vi "CheckTracepoint.vi"(8 "error in (no error)":errorcluster, 11 "tracepoint":string) -> (0 "error out":errorcluster, 1 "found":bool, 2 "enabled":bool)   [LabVIEW 2017, in "TraceLogger.lvlib"]
uses:
  <vilib>/addons/TraceLogger/TraceLogger.lvlib
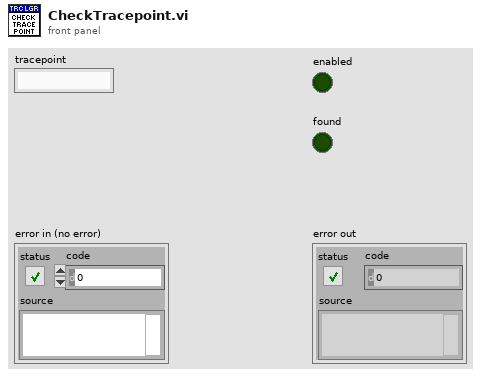
[diagram p1: front panel]
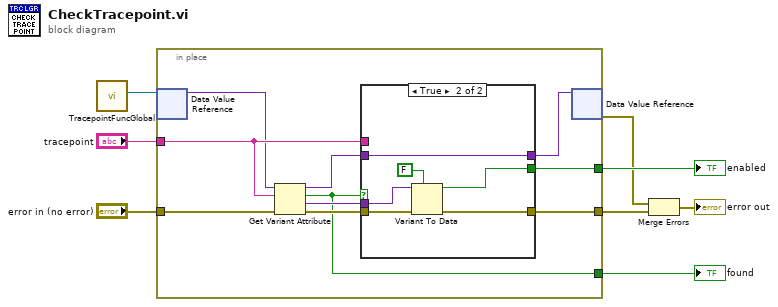
[diagram p0: block diagram]
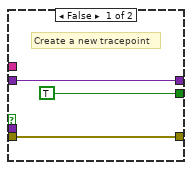
[diagram p2: hidden frame]
diagram:
  n1 = call <vilib>:"TracepointFuncGlobal.vi"() -> ("tracepoints"=w6:refnum<data-value>)  [unwired: 11 in]
  n2 = in-place {
    in-place-border: "error in (no error)" -> [w18]
    in-place-border: [w16] -> w3
    in-place-border: [w15] -> w7
    in-place-border: "tracepoint" -> [w11]
    in-place-border: [w13] -> w1
    n3 = in-place-dvr #1(w6) -> (w10:variant)  [unwired: 1 out]
    n4 = Get Variant Attribute(Variant=w10, name=w11, error in=w18) -> (duplicate Variant=w12:variant, found=w13:bool, value=w14:variant, error out=w17:errorcluster)  [unwired: 1 in]
    n5 = case shown="True" w13 {
      tunnel: w17 -> [w20 w27]
      tunnel: [w20 w23] -> w16
      tunnel: [TRUE w24] -> w15
      tunnel: w14 -> [_ w26]
      tunnel: w12 -> [w19 w22]
      tunnel: w11 -> [_ _]
      tunnel: [w19 w22] -> w9
      frame False {
        # "Create a new tracepoint"
      }
      frame True {
        n6 = Variant To Data(error in=w27, type=FALSE, Variant=w26) -> (data=w24:bool, error out=w23:errorcluster)
      }
    }
    n7 = in-place-dvr #1(w9) -> (w5:errorcluster)  [unwired: 1 out]
  }
  "enabled" <- w7
  "found" <- w1
  n8 = Merge Errors(w5, w3) -> (→"error out":errorcluster)
